vi "SendWfrm.vi"(8 "ErrorArray In":errorcluster[](array[cluster]), 10 "clFrontPanelControlRefs":T1, 11 "NISTBus In":refnum<class "NISTBus.lvclass">) -> (0 "ErrorArray Out":errorcluster[](array[cluster]), 3 "NISTBus Out":refnum<class "NISTBus.lvclass">)   [LabVIEW 2014, in "Bus.lvlib" / "NISTBus.lvclass"]
uses:
  NISTBus.lvclass
  Framework/FrontPanel/TypeDefs/clFrontPanelControlRefs.ctl
  FGenPlugins/MyPluginBaseClass/TypeDef/PluginParams.ctl
  WfrmGenerator/WfrmPlugins/EventPluginBaseClass/TypeDefs/dblEvtSignalArray.ctl
  FGenPlugins/MyPluginBaseClass/TypeDef/CreateArbWfrmParams.ctl
  WfrmGenerator/WfrmPlugins/EventPluginBaseClass/TypeDefs/clEvtConfig.ctl
  WfrmGenerator/WfrmModule/PublicAPI/Arguments/Requests/dblEvtParams.ctl
  FGenPlugins/MyPluginBaseClass/TypeDef/ConfigArbWfrmParams.ctl
  FGenPlugins/MyPluginBaseClass/TypeDef/TriggerParams.ctl
  <userlib>/NIST/NISTErrorLib/NISTErrorLib.lvlib
  FGenPlugins/MyPluginBaseClass/NISTFGenPluginsBase.lvclass
  WfrmGenerator/WfrmPlugins/EventPluginBaseClass/BaseWfrmPlugin.lvclass
  Framework/TestFramework.lvlib
  WfrmGenerator/WfrmModule/WfrmModule.lvlib
panel:
  # "When you add a control \non the front panel, add a\nreference for it in this\ntype def.  This cluster\nwill hold all of the refer-\nences to the front panel\ncontrols in order to pass\nthese control references \nto subvis."
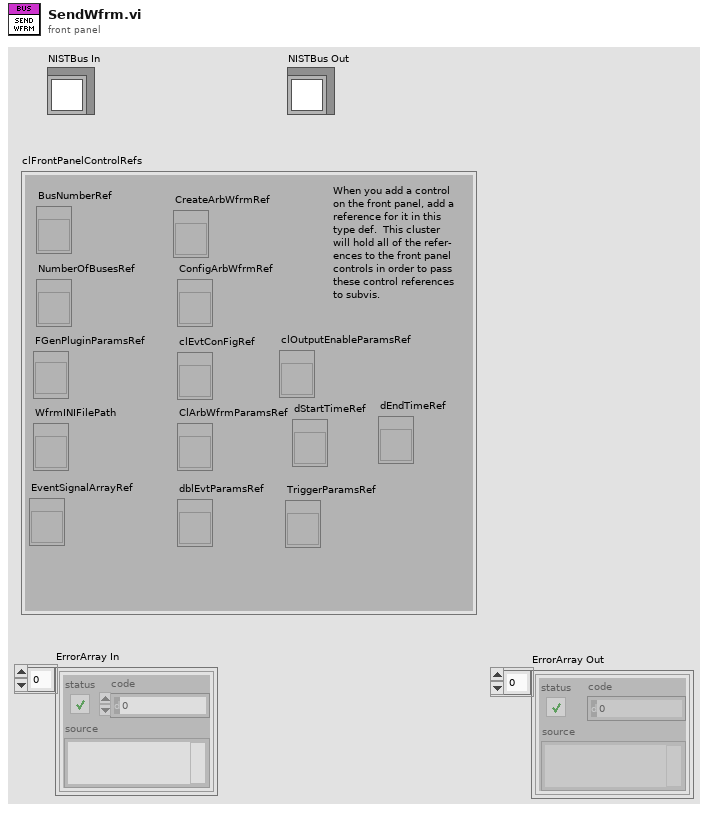
[diagram p1: front panel]
types:
  T1 = typedef "TestFramework.lvlib/clFrontPanelControlRefs.ctl" = cluster{"BusNumberRef":refnum<vi>, "NumberOfBusesRef":refnum<vi>, "FGenPluginParamsRef":refnum<vi>, "WfrmINIFilePath":refnum<vi>, "EventSignalArrayRef":refnum<vi>, "CreateArbWfrmRef":refnum<vi>, "clEvtConFigRef":refnum<vi>, "dblEvtParamsRef":refnum<vi>, "clOutputEnableParamsRef":refnum<vi>, "ConfigArbWfrmRef":refnum<vi>, "ClArbWfrmParamsRef":refnum<vi>, "dStartTimeRef":refnum<vi>, "dEndTimeRef":refnum<vi>, "TriggerParamsRef":refnum<vi>}
  T2 = cluster{"Handle":refnum<visa-resource-name>, "sName":string, "iSize":i32, "dData":dbl[], "sWfrmHandle":string}
  T3 = typedef "NISTWfrmPlugins.lvlib/EventPluginBaseClass.lvclass/dblEvtSignalArray.ctl" = dbl[][]
  T4 = typedef "NISTFGenPlugins.lvlib/NISTFGenPluginsBase.lvclass/CreateArbWfrmParams.ctl" = cluster{"sName":string, "iSize":i32, "dData":dbl[], "sWfrmHandle":string}
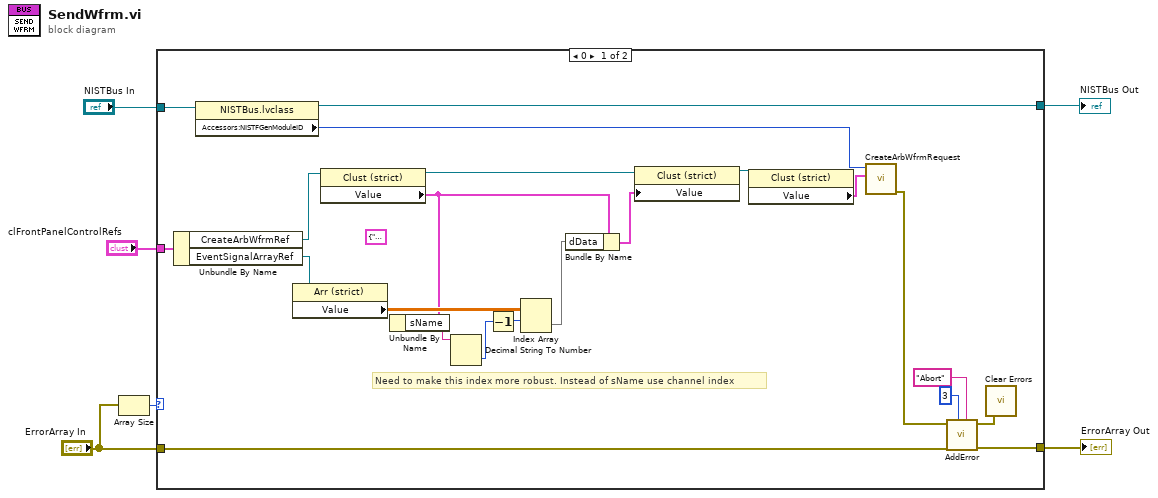
[diagram p0: block diagram]
diagram:
  n1 = Array Size(array="ErrorArray In") -> (size(s)=w6:i32)
  n2 = case shown="0" w6 {
    tunnel: "ErrorArray In" -> [w25 w30]
    tunnel: [w24 w30] -> w4
    tunnel: "NISTBus In" -> [w23 w29]
    tunnel: "clFrontPanelControlRefs" -> [w21 _]
    tunnel: [w22 w29] -> w1
    frame 0 {
      (unwired) T2 {"Handle"="", "sName"="", "iSize"=0, "dData"=[], "sWfrmHandle"=""} ("CreateArbWfrmParams")
      # "Need to make this index more robust. Instead of sName use channel index"
      n3 = Unbundle By Name(w21) -> ("CreateArbWfrmRef"=w20:refnum<vi>, "EventSignalArrayRef"=w19:refnum<vi>)
      n4 = property class="NISTBus.lvclass"(reference=w23) -> (reference out=w22:refnum<class "NISTBus.lvclass">, "Accessors:NISTFGenModuleID"=w17:i32)  [unwired: 1 in, 1 out]
      n5 = property class="Arr (strict)"(reference=w19) -> ("Value"=w18:T3)  [unwired: 1 in, 2 out]
      n6 = property class="Clust (strict)"(reference=w20) -> (reference out=w13:refnum<vi>, "Value"=w10:T4)  [unwired: 1 in, 1 out]
      n7 = Unbundle By Name(w10) -> ("sName"=w9:string)
      n8 = Decimal String To Number(string=w9) -> (number=w7:i32)  [unwired: 2 in, 1 out]
      n9 = Decrement(x=w7) -> (x-1=w8:i32)
      n10 = Index Array(array=w18, index (row)=w8) -> (element=w14:dbl[])  [unwired: 1 in]
      n11 = Bundle By Name(cluster=w10, "dData"=w14) -> (w11:T4)
      n12 = property class="Clust (strict)"(reference=w13, "Value"=w11) -> (reference out=w12:refnum<vi>)  [unwired: 1 in, 1 out]
      n13 = property class="Clust (strict)"(reference=w12) -> ("Value"=w16:T4)  [unwired: 1 in, 2 out]
      n14 = call "CreateArbWfrmRequest.vi"("CreateArbWfrmParams"=w16, "ModuleID"=w17) -> ("error out"=w15:errorcluster)  [unwired: 9 in]
      n15 = call <userlib>:"AddError.vi"("Severity"="Abort" ("String"), "Priority"=u8 3, "ErrorArray"=w25, "error in (no error)"=w15) -> ("ErrorArray"=w24:errorcluster[], "error out"=w26:errorcluster)  [unwired: 6 in]
      n16 = call <vilib>:"Clear Errors.vi"("error in (no error)"=w26) -> ()  [unwired: 5 in, 2 out]
    }
    frame 1, Default {
    }
  }
  "NISTBus Out" <- w1
  "ErrorArray Out" <- w4
